vi "AWG Write Multiple Standard Waveforms From File.vi"(6 "SourceFolder Path":string, 8 "error in (no error)":errorcluster, 9 "AmpGain":i32=1, 10 "Channel Configurations":T2(array[cluster])=[{"PinNames"=["UP"], "WaveFormFile Name"=""}, {"PinNames"=["DOWN"], "WaveFormFile Name"=""}], 11 "Semiconductor Module Context":T1) -> (0 "error out":errorcluster)   [LabVIEW 2013]
uses:
  <vilib>/NI_TestStand_SemiconductorModule/NI_TestStand_Semiconductor_Module.lvlibp/PinMap/General/SemiconductorModuleContext.ctl
  <instrlib>/niFgen/niFgen.llb/niFgen Write Named Waveform (I16).vi
  <vilib>/NI_TestStand_SemiconductorModule/NI_TestStand_Semiconductor_Module.lvlibp
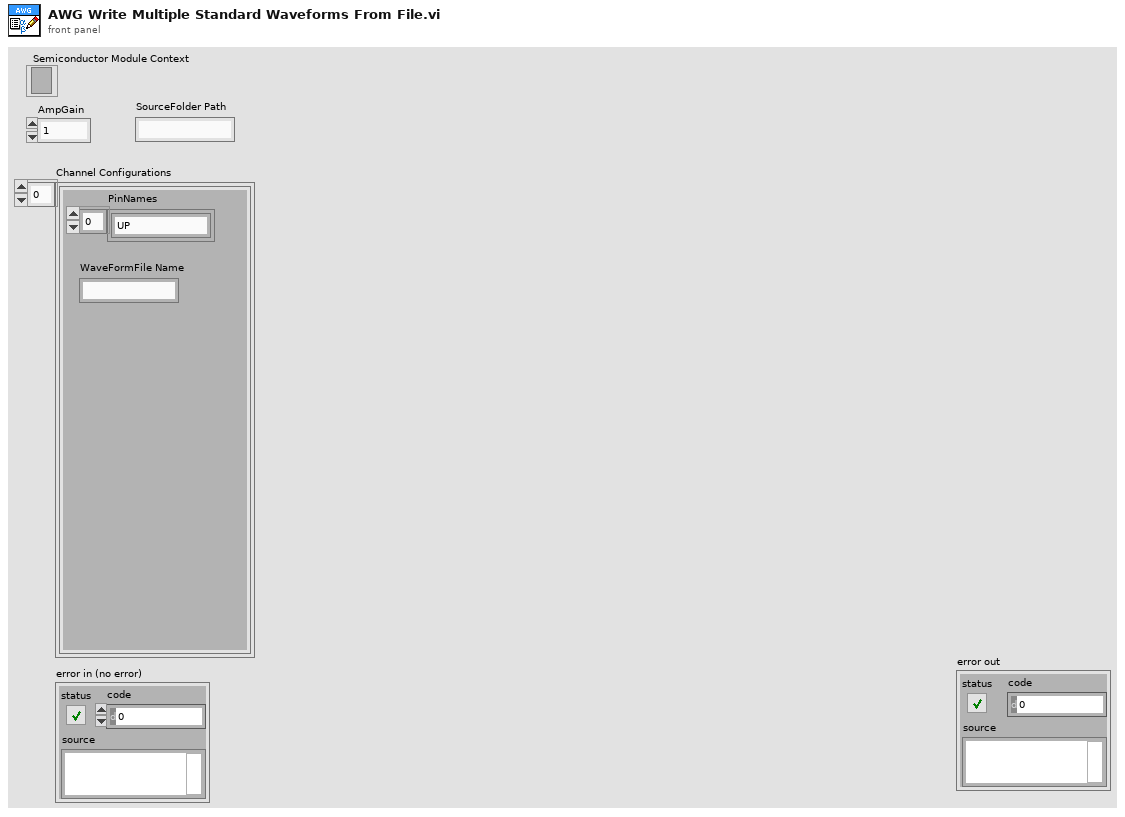
[diagram p1: front panel]
types:
  T1 = typedef "NI_TestStand_Semiconductor_Module.lvlibp/SemiconductorModuleContext.ctl" = refnum<k7>
  T2 = cluster{"PinNames":string[], "WaveFormFile Name":string}[]
  T3 = typedef "StandardWaveformWithName.ctl" = cluster{"Name":string, "Waveform":T4}
  T4 = typedef "StandardWaveform.ctl" = cluster{"waveform type":enum16{"sine", "cosine", "triangle", "square", "sawtooth", "increasing ramp", "decreasing ramp", "DC Value"}, "amplitude":dbl, "Time":dbl}
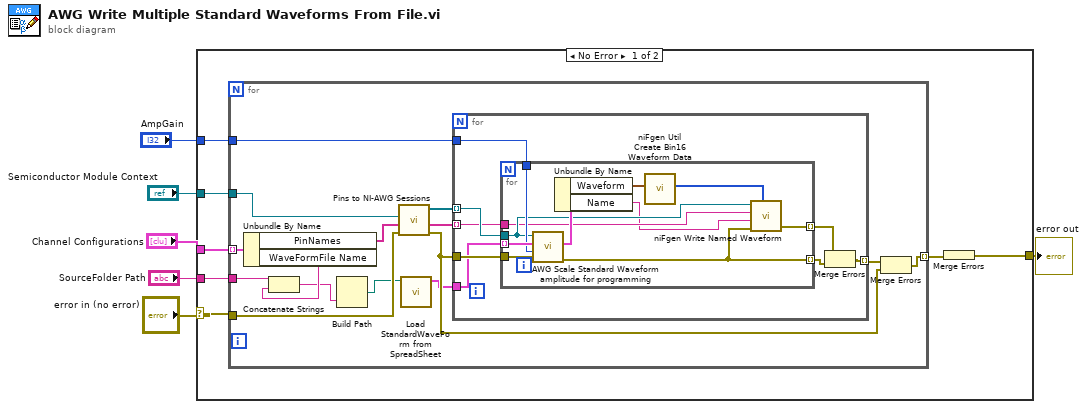
[diagram p0: block diagram]
diagram:
  n1 = case shown="No Error" "error in (no error)" {
    selector: "error in (no error)" -> [w9 w48]
    tunnel: "Channel Configurations" -> [w13 _]
    tunnel: "Semiconductor Module Context" -> [w12 _]
    tunnel: [w10 w48] -> w4
    tunnel: "AmpGain" -> [w8 _]
    tunnel: "SourceFolder Path" -> [w7 _]
    frame No Error {
      n2 = for {
        tunnel: [w23] -> w11 mode=indexing
        tunnel: w13 -> [w26] mode=indexing
        tunnel: w9 -> [w25]
        tunnel: w12 -> [w24]
        tunnel: w8 -> [w21]
        tunnel: w7 -> [w17]
        n3 = Unbundle By Name(w26) -> ("PinNames"=w22:string[], "WaveFormFile Name"=w16:string)
        n4 = Concatenate Strings(w17, w16) -> (w14:string)
        n5 = Build Path(name or relative path=w14) -> (appended path=w15:path)  [unwired: 1 in]
        n6 = call "Pins to NI-AWG Sessions.vi"("error in (no error)"=w25, "Pins"=w22, "Semiconductor Module Context"=w24) -> ("error out"=w20:errorcluster, "Channel Lists"=w27:string[], "Instrument Sessions"=w28:refnum<k15>[])  [unwired: 5 in, 1 out]
        n7 = call "Load StandardWaveForm from SpreadSheet.vi"("Path"=w15) -> ("StandardWaveforms Array"=w18:T3[])  [unwired: 10 in]
        n8 = for {
          tunnel: w20 -> [w36]
          tunnel: w18 -> [w35]
          tunnel: w28 -> [w33] mode=indexing
          tunnel: w27 -> [w29] mode=indexing
          tunnel: w21 -> [w34]
          tunnel: [w31] -> w19 mode=indexing
          n9 = for {
            tunnel: w36 -> [w47]
            tunnel: [w41] -> w32 mode=indexing
            tunnel: w33 -> [w39]
            tunnel: w35 -> [w46] mode=indexing
            tunnel: w34 -> [w45]
            tunnel: [w42] -> w30 mode=indexing
            tunnel: w29 -> [w38]
            n10 = call "AWG Scale Standard Waveform amplitude for programming.vi"("error in (no error)"=w47, "AmpGain"=w45, "Waveform In"=w46, "Instrument Handle In"=w39) -> ("error out"=w41:errorcluster, "Waveform Out"=w44:T3)  [unwired: 5 in, 1 out]
            n11 = Unbundle By Name(w44) -> ("Waveform"=w43:T4, "Name"=w37:string)
            n12 = call <instrlib>:"niFgen Util Create Bin16 Waveform Data.vi"("Waveform"=w43) -> ("Waveform Data"=w40:i16[])  [unwired: 10 in]
            n13 = call-poly <instrlib>:"niFgen Write Named Waveform.vi"("Waveform Data"=w40, "error in (no error)"=w41, "Waveform Name"=w37, "Channel Name"=w38, "Instrument Handle"=w39) -> ("error out"=w42:errorcluster)  [unwired: 4 in, 2 out]
          }
          n14 = Merge Errors(w30, w32) -> (w31:errorcluster)
        }
        n15 = Merge Errors(w19, w20) -> (w23:errorcluster)
      }
      n16 = Merge Errors(w11) -> (w10:errorcluster)
    }
    frame Error {
    }
  }
  "error out" <- w4
